vi "WPI_SerialPortCoiteratedSort.vi"(10 "Array to Sort":string[](array[string]), 11 "Coiterated Array":string[](array[string])) -> (2 "Sorted Array":string[](array[string]), 3 "Coiterated Array Out":string[](array[string]))   [LabVIEW 2017]
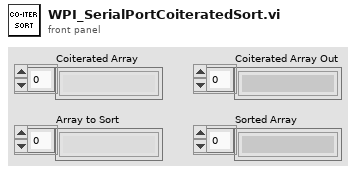
[diagram p1: front panel]
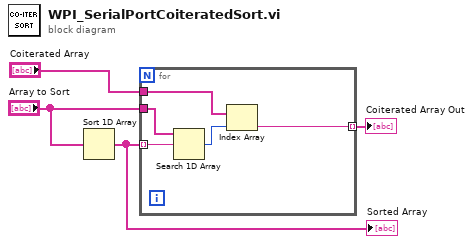
[diagram p0: block diagram]
diagram:
  n1 = Sort 1D Array(array="Array to Sort") -> (sorted array=w1:string[])
  "Sorted Array" <- w1
  n2 = for {
    tunnel: w1 -> [w8] mode=indexing
    tunnel: "Array to Sort" -> [w9]
    tunnel: "Coiterated Array" -> [w6]
    tunnel: [w5] -> w4 mode=indexing
    n3 = Search 1D Array(1D array=w9, element=w8) -> (index of element=w7:i32)  [unwired: 1 in]
    n4 = Index Array(array=w6, index=w7) -> (element=w5:string)
  }
  "Coiterated Array Out" <- w4
